vi "FGV-BroadcastRegistry.vi"(0 "Source":string, 5 "Target":string, 7 "Message":string, 9 "Response Message In":string, 11 "Error in":errorcluster caption="Error in (no error)", 12 "Operation":T2, 13 "Priority":T1) -> (4 "Response Message Info":T3, 8 "Cluster":cluster{"Registry":variant}, 15 "Error out":errorcluster)   [LabVIEW 2014, in "JKI State Machine++.lvlib"]
uses:
  JKI State Machine++.lvlib
  Typedef/_JKISM_Broadcast_Response_Message_info.ctl
  AdvanceAPI/JKISM++ Broadcast Message Type.ctl
  Operation-BroadcastRegistry.ctl
  global-Broadcast Cache Change Flag.vi
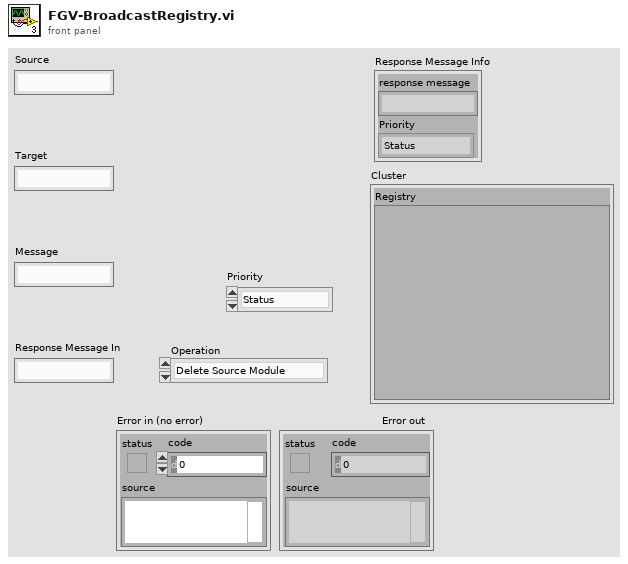
[diagram p1: front panel]
types:
  T1 = typedef "JKI State Machine++.lvlib/JKISM++ Broadcast Message Type.ctl" = enum16{"Status", "Interrupt(High)"}
  T2 = typedef "JKI State Machine++.lvlib/Operation-BroadcastRegistry.ctl" = enum16{"Delete Source Module", "Delete Target Module", "Remove Module", "Register", "Unregister", "Check"}
  T3 = typedef "JKI State Machine++.lvlib/_JKISM_Broadcast_Response_Message_info.ctl" = cluster{"response message":string, "Priority":T1}
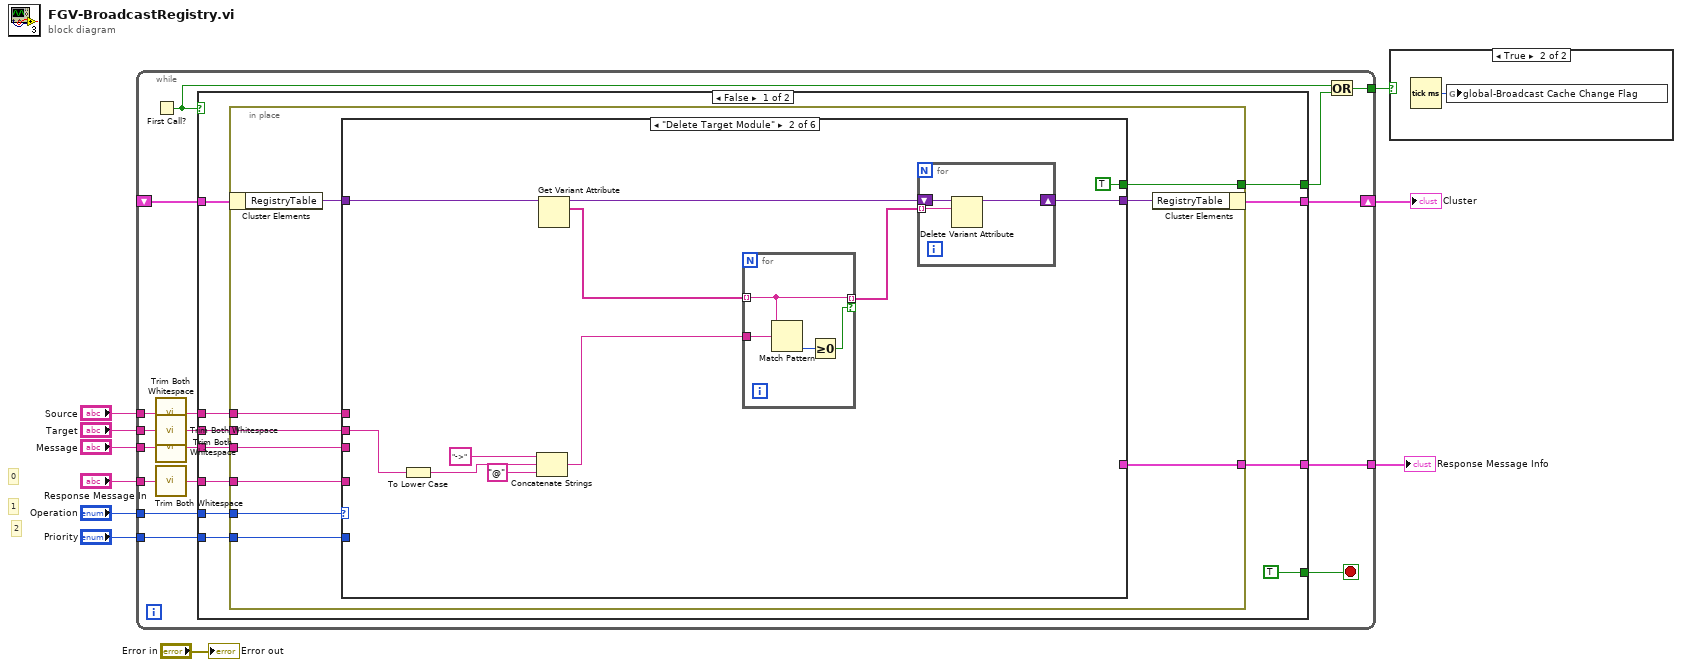
[diagram p0: block diagram]
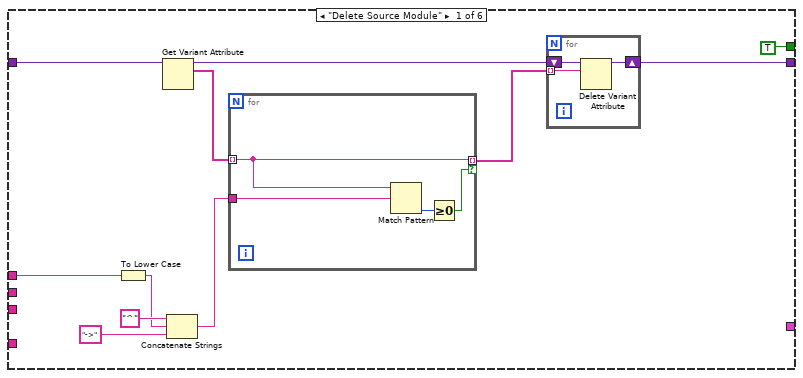
[diagram p3: hidden frame]
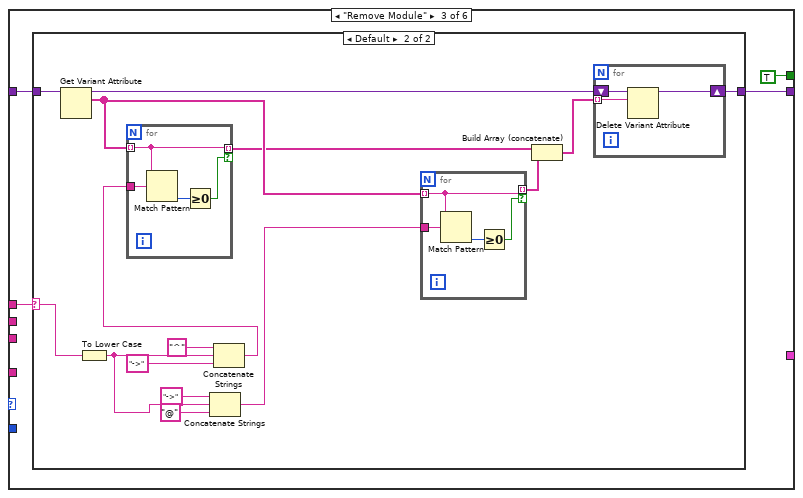
[diagram p4: hidden frame]
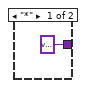
[diagram p5: hidden frame]
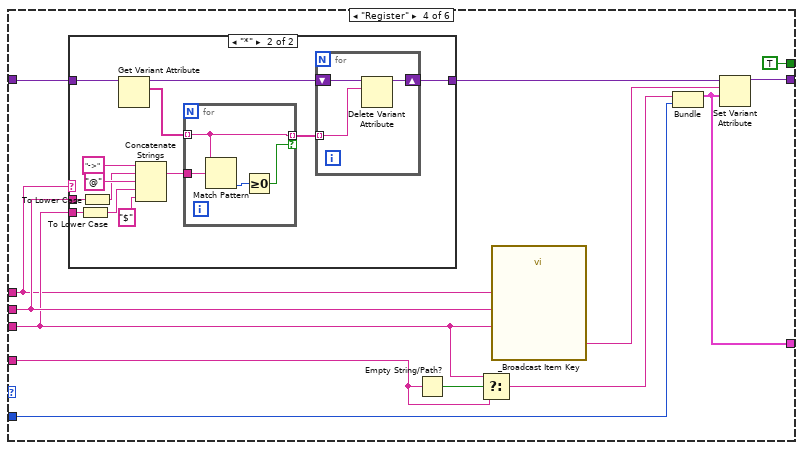
[diagram p6: hidden frame]
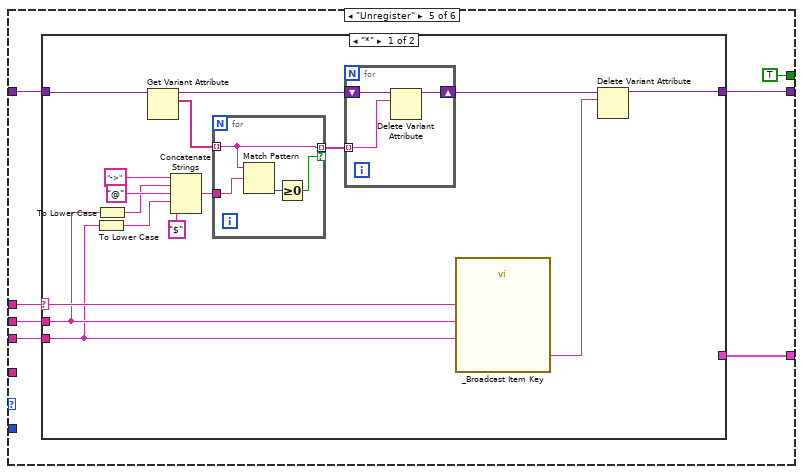
[diagram p8: hidden frame]
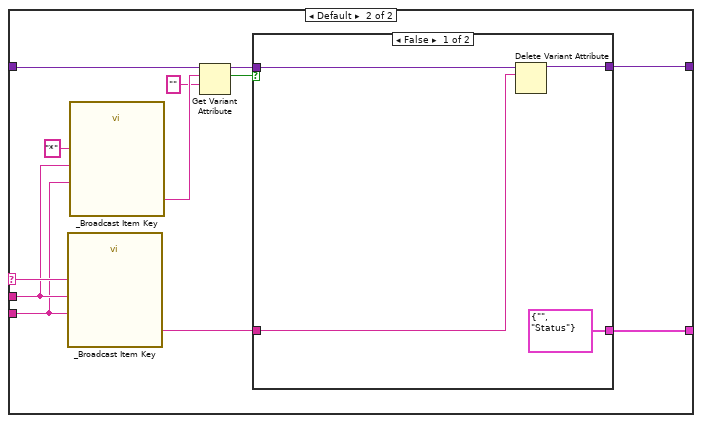
[diagram p9: hidden frame]
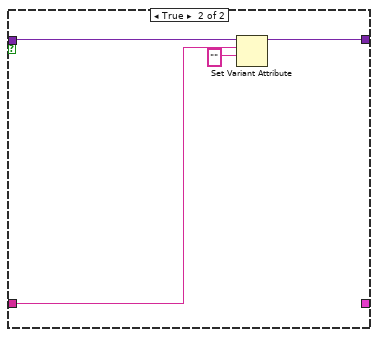
[diagram p10: hidden frame]
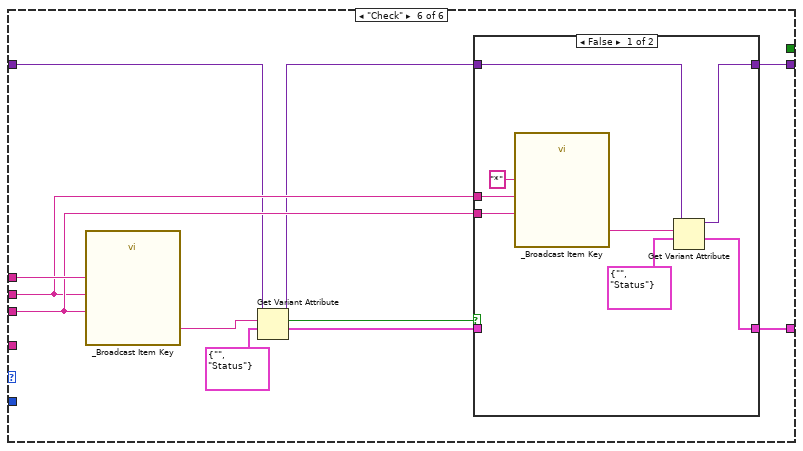
[diagram p11: hidden frame]
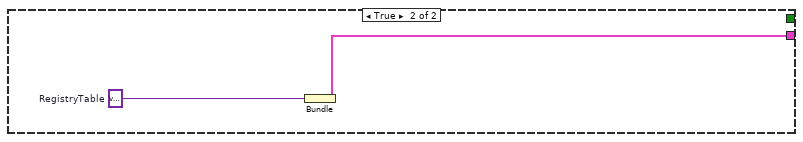
[diagram p13: hidden frame]
diagram:
  # "2"
  # "0"
  # "1"
  n1 = while {
    shift-right: [w26] -> w2
    shift-left: _ -> [w25]
    tunnel: "Operation" -> [w24]
    tunnel: "Target" -> [w17]
    tunnel: "Source" -> [w16]
    tunnel: "Message" -> [w18]
    tunnel: "Response Message In" -> [w19]
    tunnel: [w23] -> w5
    tunnel: [w20] -> w3
    tunnel: "Priority" -> [w11]
    stop <- w27 stop-if-true
    n2 = First Call?() -> (First Call?: T/F=w21:bool)
    n3 = call "Trim Both Whitespace.vi"("string"=w16) -> ("trimmed string"=w15:string)  [unwired: 1 in]
    n4 = call "Trim Both Whitespace.vi"("string"=w17) -> ("trimmed string"=w14:string)  [unwired: 1 in]
    n5 = call "Trim Both Whitespace.vi"("string"=w18) -> ("trimmed string"=w13:string)  [unwired: 1 in]
    n6 = call "Trim Both Whitespace.vi"("string"=w19) -> ("trimmed string"=w12:string)  [unwired: 1 in]
    n7 = case shown="False" w21 {
      tunnel: [TRUE _] -> w27
      tunnel: [w36 w221] -> w26
      tunnel: w25 -> [w37 _]
      tunnel: w24 -> [w35 _]
      tunnel: w14 -> [w34 _]
      tunnel: w15 -> [w33 _]
      tunnel: w13 -> [w32 _]
      tunnel: w12 -> [w31 _]
      tunnel: [w30 _] -> w23
      tunnel: [w29 _] -> w22
      tunnel: w11 -> [w28 _]
      frame False {
        n8 = in-place {
          in-place-border: w35 -> [w48]
          in-place-border: w34 -> [w45]
          in-place-border: w33 -> [w44]
          in-place-border: w32 -> [w43]
          in-place-border: w31 -> [w42]
          in-place-border: [w41] -> w30
          in-place-border: [w40] -> w29
          in-place-border: w28 -> [w39]
          n9 = in-place-cluster #1(w37) -> ("RegistryTable"=w46:variant)
          n10 = case shown="\"Delete Target Module\"" w48 {
            tunnel: [w58 w75 w88 w128 w154 w204] -> w47
            tunnel: w46 -> [w57 w73 w87 w122 w155 w206]
            tunnel: w45 -> [_ w67 _ w121 w151 w207]
            tunnel: w44 -> [w49 _ w85 w118 w156 w209]
            tunnel: w43 -> [_ _ _ w119 w150 w208]
            tunnel: w42 -> [_ _ _ w127 _ _]
            tunnel: [_ _ _ w116 w153 w201] -> w41
            tunnel: [TRUE ("Cache changed?") TRUE ("Cache changed?") TRUE ("Cache changed?") TRUE ("Cache changed?") TRUE ("Cache changed?") _] -> w40
            tunnel: w39 -> [_ _ _ w117 _ _]
            frame "Delete Source Module" {
              n11 = To Lower Case(string=w49) -> (all lower case string=w50:string)
              n12 = Get Variant Attribute(Variant=w57) -> (duplicate Variant=w56:variant, names=w55:string[])  [unwired: 3 in, 2 out]
              n13 = Concatenate Strings("^" ("string"), w50, "->" ("string")) -> (w52:string)
              n14 = for {
                tunnel: w55 -> [w66] mode=indexing
                tunnel: [w66] -> w54 mode=indexing if=w63
                tunnel: w52 -> [w65]
                n15 = Match Pattern(string=w66, regular expression=w65) -> (offset past match=w64:i32)  [unwired: 1 in, 3 out]
                n16 = Greater Or Equal To 0?(x=w64) -> (x >= 0?=w63:bool)
              }
              n17 = for {
                tunnel: w54 -> [w60] mode=indexing
                shift-right: [w62] -> w58
                shift-left: w56 -> [w61]
                n18 = Delete Variant Attribute(6:w60, 7:w61) -> (3:w62:variant)  [unwired: 1 in, 2 out]
              }
            }
            frame "Delete Target Module" {
              n19 = To Lower Case(string=w67) -> (all lower case string=w74:string)
              n20 = Concatenate Strings("->" ("string"), w74, "@" ("string")) -> (w69:string)
              n21 = Get Variant Attribute(Variant=w73) -> (duplicate Variant=w72:variant, names=w71:string[])  [unwired: 3 in, 2 out]
              n22 = for {
                tunnel: w71 -> [w84] mode=indexing
                tunnel: [w84] -> w70 mode=indexing if=w81
                tunnel: w69 -> [w83]
                n23 = Match Pattern(string=w84, regular expression=w83) -> (offset past match=w82:i32)  [unwired: 1 in, 3 out]
                n24 = Greater Or Equal To 0?(x=w82) -> (x >= 0?=w81:bool)
              }
              n25 = for {
                tunnel: w70 -> [w78] mode=indexing
                shift-right: [w80] -> w75
                shift-left: w72 -> [w79]
                n26 = Delete Variant Attribute(6:w78, 7:w79) -> (3:w80:variant)  [unwired: 1 in, 2 out]
              }
            }
            frame "Remove Module" {
              n27 = case shown="Default" w85 {
                selector: w85 -> [_ w90]
                tunnel: [variant w103] -> w88
                tunnel: w87 -> [_ w102]
                frame "*" {
                }
                frame Default {
                  n28 = Get Variant Attribute(Variant=w102) -> (duplicate Variant=w101:variant, names=w98:string[])  [unwired: 3 in, 2 out]
                  n29 = To Lower Case(string=w90) -> (all lower case string=w95:string)
                  n30 = Concatenate Strings("->" ("string"), w95, "@" ("string")) -> (w93:string)
                  n31 = Concatenate Strings("^" ("string"), w95, "->" ("string")) -> (w94:string)
                  n32 = for {
                    tunnel: w98 -> [w108] mode=indexing
                    tunnel: [w108] -> w91 mode=indexing if=w106
                    tunnel: w94 -> [w105]
                    n33 = Match Pattern(string=w108, regular expression=w105) -> (offset past match=w107:i32)  [unwired: 1 in, 3 out]
                    n34 = Greater Or Equal To 0?(x=w107) -> (x >= 0?=w106:bool)
                  }
                  n35 = for {
                    tunnel: w98 -> [w115] mode=indexing
                    tunnel: [w115] -> w100 mode=indexing if=w112
                    tunnel: w93 -> [w114]
                    n36 = Match Pattern(string=w115, regular expression=w114) -> (offset past match=w113:i32)  [unwired: 1 in, 3 out]
                    n37 = Greater Or Equal To 0?(x=w113) -> (x >= 0?=w112:bool)
                  }
                  n38 = Build Array (concatenate)(w91, w100) -> (w92:string[])
                  n39 = for {
                    tunnel: w92 -> [w109] mode=indexing
                    shift-right: [w111] -> w103
                    shift-left: w101 -> [w110]
                    n40 = Delete Variant Attribute(6:w109, 7:w110) -> (3:w111:variant)  [unwired: 1 in, 2 out]
                  }
                }
              }
            }
            frame "Register" {
              n41 = case shown="\"*\"" w118 {
                tunnel: w122 -> [w129 w142]
                tunnel: w121 -> [_ w135]
                tunnel: [w129 w134] -> w120
                tunnel: w119 -> [_ w132]
                frame Default {
                }
                frame "*" {
                  n42 = To Lower Case(string=w132) -> (all lower case string=w131:string)
                  n43 = To Lower Case(string=w135) -> (all lower case string=w137:string)
                  n44 = Get Variant Attribute(Variant=w142) -> (duplicate Variant=w141:variant, names=w140:string[])  [unwired: 3 in, 2 out]
                  n45 = Concatenate Strings("->" ("string"), w137, "@" ("string"), w131, "$" ("string")) -> (w136:string)
                  n46 = for {
                    tunnel: w140 -> [w149] mode=indexing
                    tunnel: [w149] -> w133 mode=indexing if=w147
                    tunnel: w136 -> [w146]
                    n47 = Match Pattern(string=w149, regular expression=w146) -> (offset past match=w148:i32)  [unwired: 1 in, 3 out]
                    n48 = Greater Or Equal To 0?(x=w148) -> (x >= 0?=w147:bool)
                  }
                  n49 = for {
                    shift-right: [w144] -> w134
                    shift-left: w141 -> [w145]
                    tunnel: w133 -> [w143] mode=indexing
                    n50 = Delete Variant Attribute(6:w143, 7:w145) -> (3:w144:variant)  [unwired: 1 in, 2 out]
                  }
                }
              }
              n51 = Empty String/Path?(string/path=w127) -> (empty?=w125:bool)
              n52 = Select(t=w119, s=w125, f=w127) -> (s? t:f=w124:string)
              n53 = call "_Broadcast Item Key.vi"("Message"=w119, "Target"=w121, "Source"=w118) -> ("Key"=w123:string)  [unwired: 2 in]
              n54 = Bundle("trimmed string"=w124, "Priority"=w117) -> (w116:cluster{"trimmed string":string, "Priority":T1})  [unwired: 1 in]
              n55 = Set Variant Attribute(Variant=w120, name=w123, value=w116) -> (Variant out=w128:variant)  [unwired: 1 in, 2 out]
            }
            frame "Unregister" {
              n56 = case shown="\"*\"" w156 {
                selector: w156 -> [w172 w183]
                tunnel: w155 -> [w162 w188]
                tunnel: [w171 w191] -> w154
                tunnel: [_ w190] -> w153
                tunnel: w151 -> [w160 w182]
                tunnel: w150 -> [w159 w181]
                frame "*" {
                  n57 = To Lower Case(string=w159) -> (all lower case string=w163:string)
                  n58 = To Lower Case(string=w160) -> (all lower case string=w165:string)
                  n59 = Get Variant Attribute(Variant=w162) -> (duplicate Variant=w169:variant, names=w168:string[])  [unwired: 3 in, 2 out]
                  n60 = Concatenate Strings("->" ("string"), w165, "@" ("string"), w163, "$" ("string")) -> (w157:string)
                  n61 = for {
                    tunnel: w168 -> [w179] mode=indexing
                    tunnel: [w179] -> w164 mode=indexing if=w176
                    tunnel: w157 -> [w178]
                    n62 = Match Pattern(string=w179, regular expression=w178) -> (offset past match=w177:i32)  [unwired: 1 in, 3 out]
                    n63 = Greater Or Equal To 0?(x=w177) -> (x >= 0?=w176:bool)
                  }
                  n64 = for {
                    shift-right: [w174] -> w161
                    shift-left: w169 -> [w175]
                    tunnel: w164 -> [w173] mode=indexing
                    n65 = Delete Variant Attribute(6:w173, 7:w175) -> (3:w174:variant)  [unwired: 1 in, 2 out]
                  }
                  n66 = call "_Broadcast Item Key.vi"("Message"=w159, "Target"=w160, "Source"=w172) -> ("Key"=w170:string)  [unwired: 2 in]
                  n67 = Delete Variant Attribute(6:w170, 7:w161) -> (3:w171:variant)  [unwired: 1 in, 2 out]
                }
                frame Default {
                  n68 = call "_Broadcast Item Key.vi"("Message"=w181, "Target"=w182, "Source"=w183) -> ("Key"=w180:string)  [unwired: 2 in]
                  n69 = call "_Broadcast Item Key.vi"("Message"=w181, "Target"=w182, "Source"="*") -> ("Key"=w186:string)  [unwired: 2 in]
                  n70 = Get Variant Attribute(Variant=w188, name=w186, default value (empty Variant)="" ("Source")) -> (duplicate Variant=w187:variant, found=w185:bool)  [unwired: 1 in, 2 out]
                  n71 = case shown="False" w185 {
                    tunnel: [w195 w199] -> w191
                    tunnel: [T3 {"response message"="", "Priority"=enum."Status"} ("Response Message Info") _] -> w190
                    tunnel: w187 -> [w194 w198]
                    tunnel: w180 -> [w193 w197]
                    frame False {
                      n72 = Delete Variant Attribute(6:w193, 7:w194) -> (3:w195:variant)  [unwired: 1 in, 2 out]
                    }
                    frame True {
                      n73 = Set Variant Attribute(Variant=w198, name=w197, value="" ("Source")) -> (Variant out=w199:variant)  [unwired: 1 in, 2 out]
                    }
                  }
                }
              }
            }
            frame "Check" {
              n74 = call "_Broadcast Item Key.vi"("Message"=w208, "Target"=w207, "Source"=w209) -> ("Key"=w210:string)  [unwired: 2 in]
              n75 = Get Variant Attribute(Variant=w206, name=w210, default value (empty Variant)=T3 {"response message"="", "Priority"=enum."Status"} ("Response Message Info")) -> (duplicate Variant=w205:variant, found=w203:bool, value=w202:T3)  [unwired: 1 in, 1 out]
              n76 = case shown="False" w203 {
                tunnel: w208 -> [w218 _]
                tunnel: w207 -> [w217 _]
                tunnel: w205 -> [w214 w220]
                tunnel: [w213 w220] -> w204
                tunnel: w202 -> [_ w219]
                tunnel: [w212 w219] -> w201
                frame False {
                  n77 = call "_Broadcast Item Key.vi"("Message"=w218, "Target"=w217, "Source"="*") -> ("Key"=w215:string)  [unwired: 2 in]
                  n78 = Get Variant Attribute(Variant=w214, name=w215, default value (empty Variant)=T3 {"response message"="", "Priority"=enum."Status"} ("Response Message Info")) -> (duplicate Variant=w213:variant, value=w212:T3)  [unwired: 1 in, 2 out]
                }
                frame True {
                }
              }
            }
          }
          n79 = in-place-cluster #1("RegistryTable"=w47) -> (w36:cluster{"RegistryTable":variant})
        }
      }
      frame True {
        w222 = variant  # RegistryTable
        n80 = Bundle("RegistryTable"=w222) -> (w221:cluster{"RegistryTable":variant})  [unwired: 1 in]
      }
    }
    n81 = Or(x=w21, y=w22) -> (x .or. y?=w20:bool)
  }
  "Response Message Info" <- w5
  "Cluster" <- w2
  n82 = case shown="True" w3 {
    frame False {
    }
    frame True {
      n83 = Tick Count (ms)() -> (millisecond timer value=w223:u32)
      n84 = global write "global-Broadcast Cache Change Flag.vi" "global-Broadcast Cache Change Flag"(w223) -> ()
    }
  }
  "Error out" <- "Error in"
